vi "Fetch Multi Eval Meas SEM Margin All Results.vi"(8 "error in (no error)":errorcluster, 10 "Instance (1)":T2=1, 11 "VISA resource name":refnum<visa-resource-name>) -> (0 "error out":errorcluster, 1 "All Margin Results":T1 {"Minimum Positive" format="%^.3e"; "Minimum Negative" format="%^.3e"; "Average Positive" format="%^.3e"; "Average Negative" format="%^.3e"; "Current Positive" format="%^.3e"; "Current Negative" format="%^.3e"}, 2 "Reliability":i32, 3 "VISA resource name out":refnum<visa-resource-name>, 5 "Out Of Tolerance":i32)   [LabVIEW 2020, in "Rohde&Schwarz CMWXP NR FR1 Measurement.lvlib"]
doc: "Returns spectrum emission mask margin results. A negative margin indicates that the trace is located above the limit line, i.e. the limit is exceeded. Results are provided for the current, average and maximum traces. For each trace, 24 values related to the negative and positive offset frequencies of emission mask areas 1 to 12 are provided. For inactive areas, NCAP is returned.\n\nAttribute:\nRSCMWXPNRFR1M_ATTR_FETCH_MULTI_EVAL_MEAS_SEM_MARGIN_ALL_RESULTS\n\nRemote-control command:\nFETCh:NRSub:MEAS<i>:MEValuation:SEMask:MARGin:ALL?"
uses:
  <instrlib>/Rohde&Schwarz CMWXP NR FR1 Measurement/Rohde&Schwarz CMWXP NR FR1 Measurement.lvlib
  <instrlib>/Rohde&Schwarz CMWXP NR FR1 Measurement/Private/_Instance.ctl
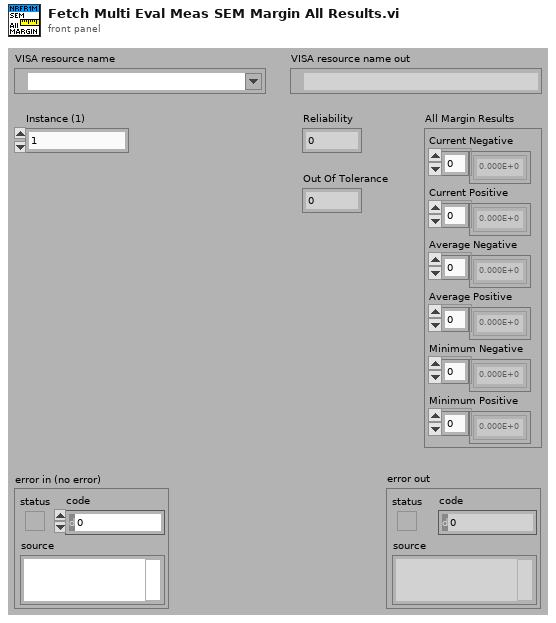
[diagram p1: front panel]
types:
  T1 = cluster{"Current Negative":dbl[], "Current Positive":dbl[], "Average Negative":dbl[], "Average Positive":dbl[], "Minimum Negative":dbl[], "Minimum Positive":dbl[]}
  T2 = typedef "Rohde&Schwarz CMWXP NR FR1 Measurement.lvlib/_Instance.ctl" = i32
  T3 = cluster{"Results":dbl[], "Results":dbl[], "Results":dbl[], "Results":dbl[], "Results":dbl[], "Results":dbl[]}
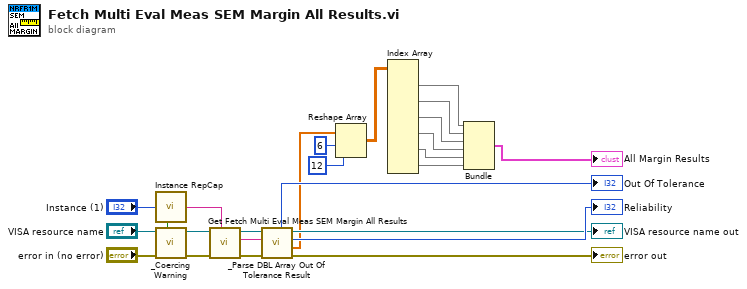
[diagram p0: block diagram]
diagram:
  n1 = call <instrlib>:"Instance RepCap.vi"("Instance In"="Instance (1)") -> ("In Range?"=w22:bool, "RepCap Identifier Out"=w21:string)  [unwired: 1 in]
  n2 = call <instrlib>:"_Coercing Warning.vi"("In Range?"=w22, "error in (no error)"="error in (no error)", "VISA resource name"="VISA resource name") -> ("error out"=w19:errorcluster, "VISA resource name out"=w20:refnum<visa-resource-name>)  [unwired: 7 in]
  n3 = call "Get Fetch Multi Eval Meas SEM Margin All Results"("Repeated Capabilities"=w21, "error in (no error)"=w19, "instrument handle"=w20) -> ("error out"=w18:errorcluster, "Fetch Multi Eval Meas SEM Margin All Results"=w16:string, "instrument handle out"=w17:refnum<visa-resource-name>)  [unwired: 6 in]
  n4 = call <instrlib>:"_Parse DBL Array Out Of Tolerance Result.vi"("error in (no error)"=w18, "Input String"=w16, "VISA resource name"=w17) -> ("error out"=→"error out":errorcluster, "Results"=w9:dbl[], "Reliability"=→"Reliability":i32, "VISA resource name out"=→"VISA resource name out":refnum<visa-resource-name>, "Out Of Tolerance"=→"Out Of Tolerance":i32)  [unwired: 4 in]
  n5 = Reshape Array(w9, 6 ("dimension size"), 12 ("dimension size")) -> (w8:dbl[][])
  n6 = Index Array(array=w8) -> (element #1=w7:dbl[], element #2=w2:dbl[], element #3=w3:dbl[], element #4=w4:dbl[], element #5=w5:dbl[], element #6=w6:dbl[])  [unwired: 12 in]
  n7 = Bundle("Results"=w7, "Results"=w2, "Results"=w3, "Results"=w4, "Results"=w5, "Results"=w6) -> (→"All Margin Results":T3)  [unwired: 1 in]
